vi "Client - JKI SM or SMO.vi"(5 "State Machine Type":enum16{"SMO", "Stand Alone"}(ring)=enum."Stand Alone", 7 "Address":string, 8 "error in (no error)":errorcluster, 11 "RemoteControl":refnum<class "RemoteControl.lvclass">) -> (0 "error out":errorcluster, 3 "RemoteControl out":refnum<class "RemoteControl.lvclass">)   [LabVIEW 2016, in "RemoteControl.lvclass"]
uses:
  RemoteControl.lvclass
  <vilib>/JKI/JKI SMO/SMO/Typedefs/SMOState --Enum.ctl
  C:/Program Files (x86)/National Instruments/LabVIEW 2016/vi.lib/JKI/JKI SMO/SMO/SMO.lvclass
  RemoteControl.lvclass/RemoteControl.ctl
  Typedefs/PrivateEvents--RemoteControl.SendMessageToProcess.ctl
  Typedefs/Message--Cluster.ctl
  <vilib>/JKI/JKI SMO/SMO/SMO.lvclass
panel:
  out "Command out":string
  out "Data out":variant
  in  "Data":variant
  in  "Command":string
  out "# reads":i32
  out "send time":u32
  out "execution time (ms)":u32
  in  "timeout in ms (100)":i32=10
  in  "Send Message":bool
  in  "Stop":bool
  out "message backlog":i32
  out "messages received":i32
  out "messages sent":i32
  in  "Port":u32=6341
  out "SMO State":T1
  # "Client - SM or SMO"
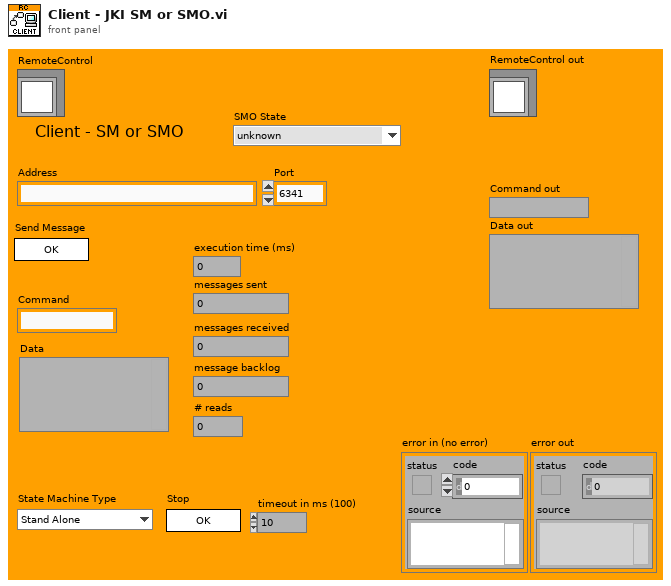
[diagram p1: front panel]
types:
  T1 = typedef "SMO.lvclass/SMOState --Enum.ctl" = enum16{"unknown", "Created", "Started", "Stopped"}
  T2 = enum32{"Invalid", "Standard", "Closed", "Hidden", "Minimized", "Maximized"}
  T3 = enum32{"invalid app kind", "Development System", "Run Time System", "Student Edition", "Embedded LabVIEW", "Evaluation", "Custom"}
  T4 = typedef "RemoteControl.lvclass/PrivateEvents--RemoteControl.SendMessageToProcess.ctl" = cluster{"Message":T5}
  T5 = typedef "RemoteControl.lvclass/Message--Cluster.ctl" = cluster{"Command":string, "Data":variant, "Message ID":i32}
  T6 = cluster{"Core":cluster{"Current VI Reference":refnum<vi>, "Close Panel on Exit?":bool}, "RemoteControl":refnum<class "RemoteControl.lvclass">}
  T7 = cluster{"Current VI Reference":refnum<vi>, "Close Panel on Exit?":bool}
  T8 = typedef "SMO.lvclass/Public Events.ctl" = cluster{"Error":refnum<user-event>, "State":refnum<user-event>, "Reserve State":refnum<user-event>}
  T9 = typedef "RemoteControl.lvclass/PublicEvents--Cluster.ctl" = cluster{"SendMessageFromProcess":refnum<user-event>}
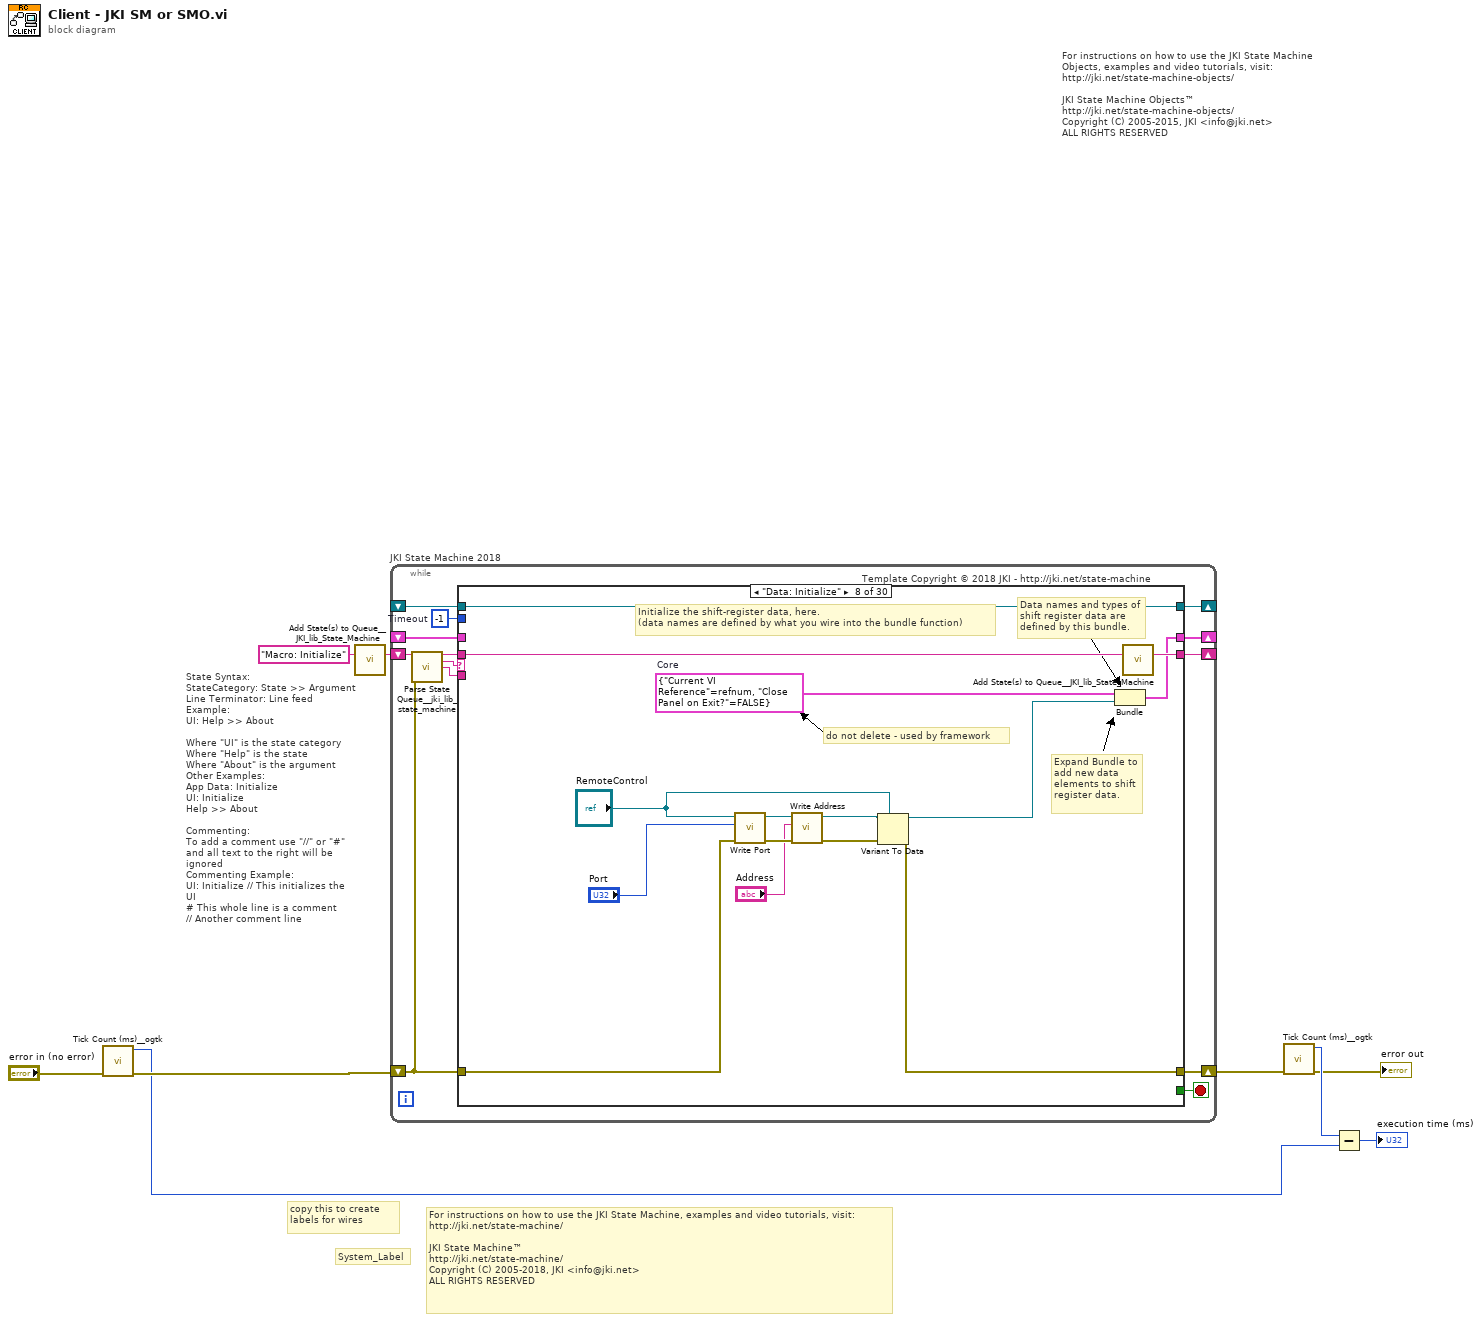
[diagram p0: block diagram]
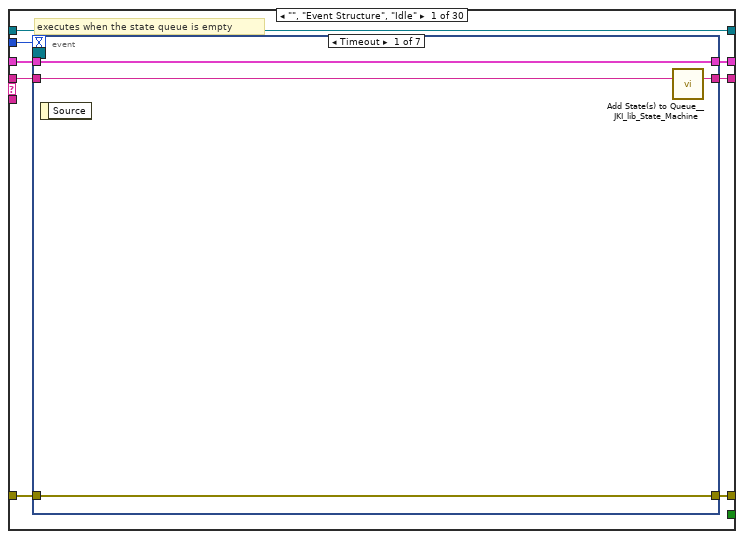
[diagram p2: hidden frame]
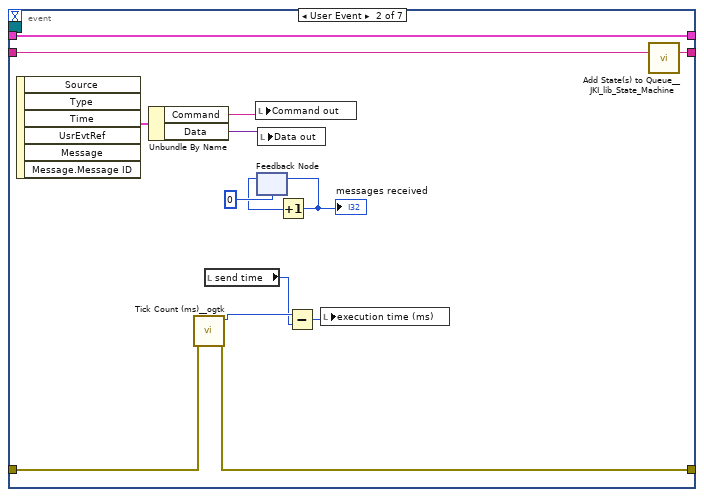
[diagram p3: hidden frame]
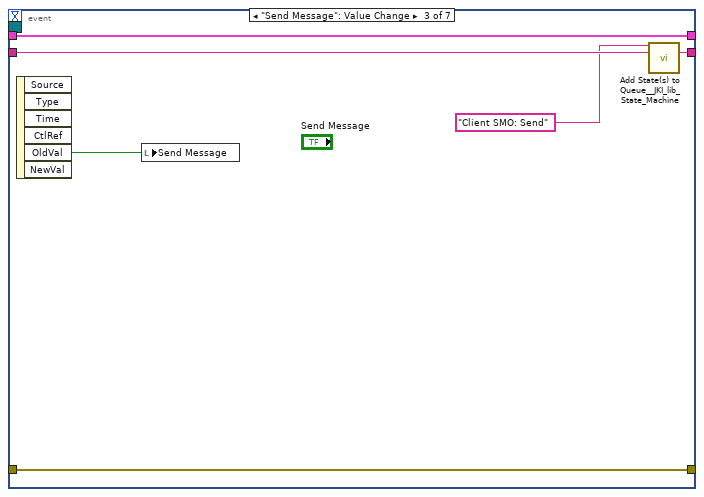
[diagram p4: hidden frame]
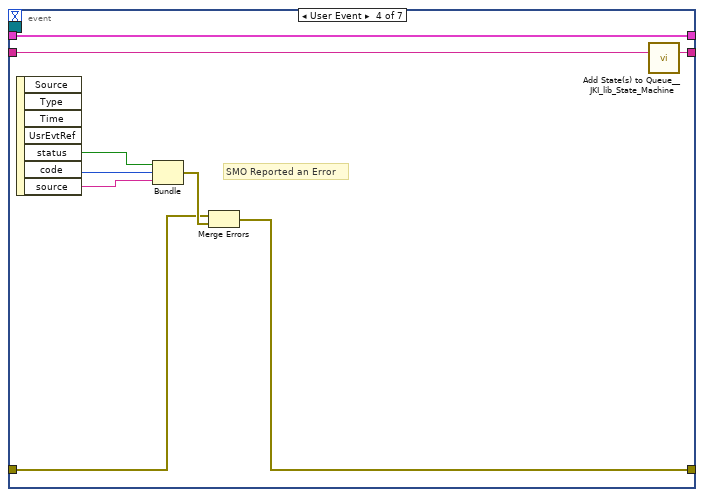
[diagram p5: hidden frame]
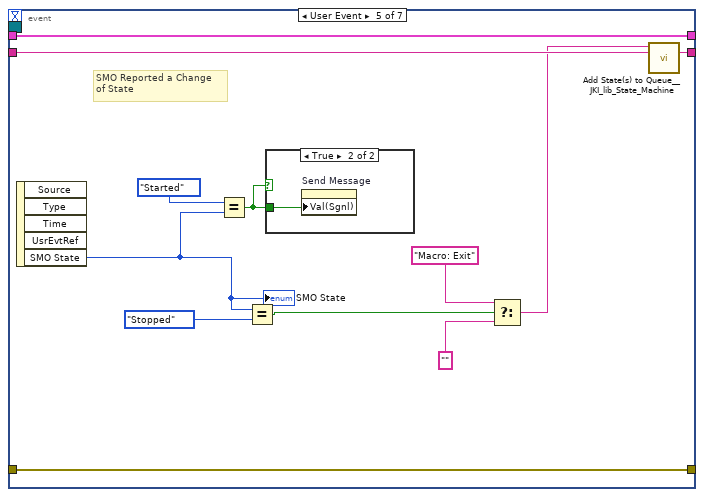
[diagram p6: hidden frame]
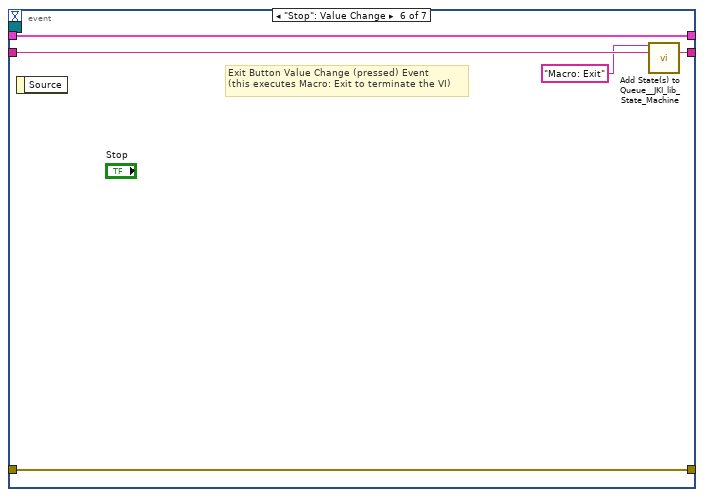
[diagram p8: hidden frame]
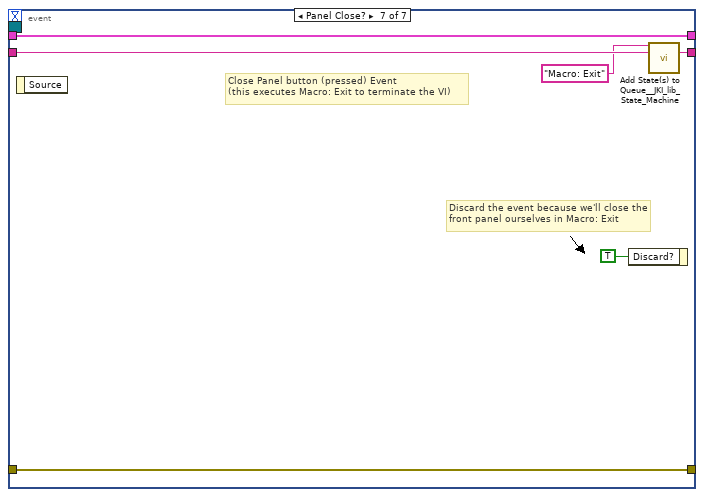
[diagram p9: hidden frame]
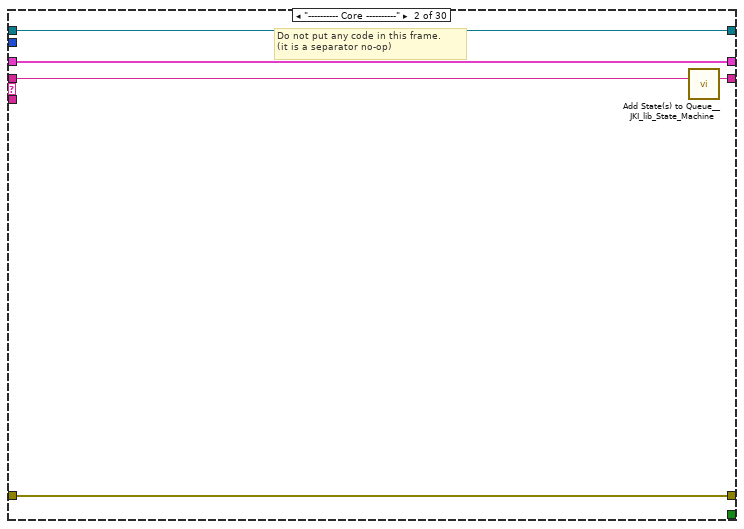
[diagram p10: hidden frame]
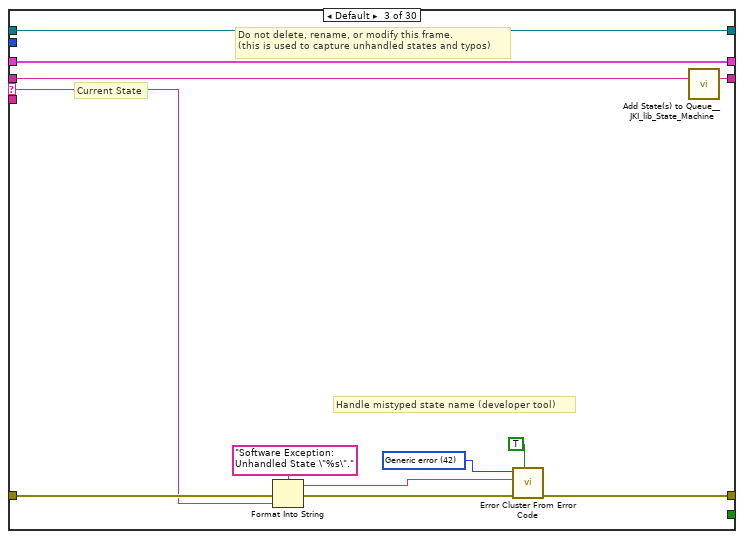
[diagram p11: hidden frame]
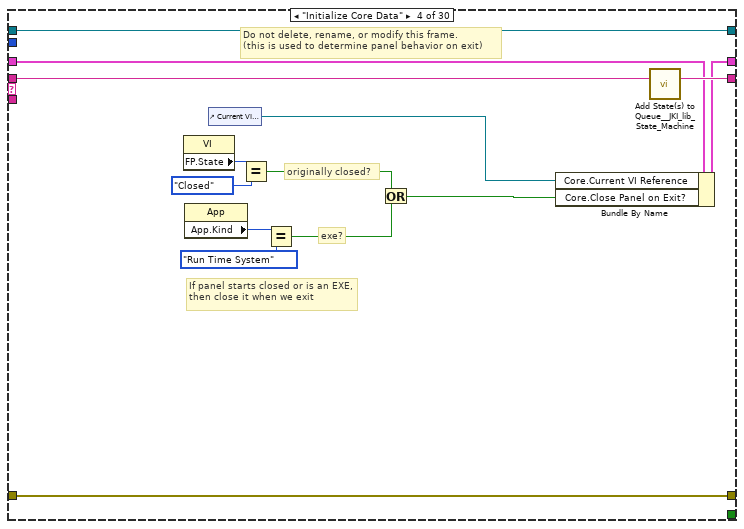
[diagram p12: hidden frame]
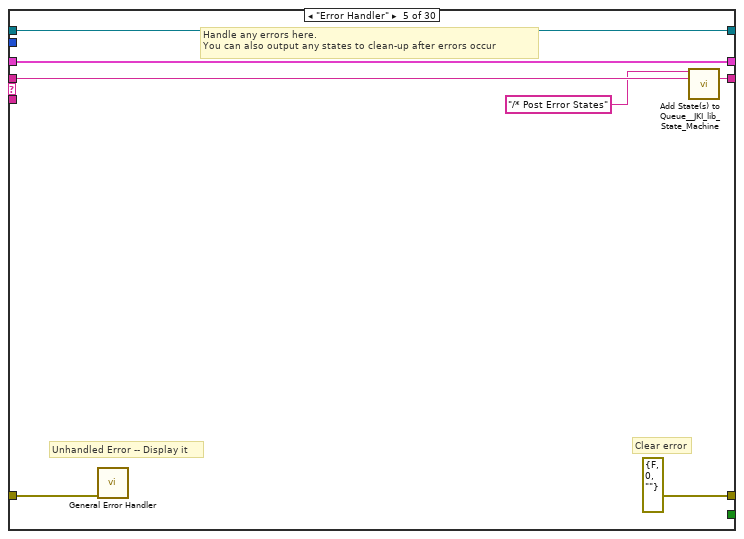
[diagram p13: hidden frame]
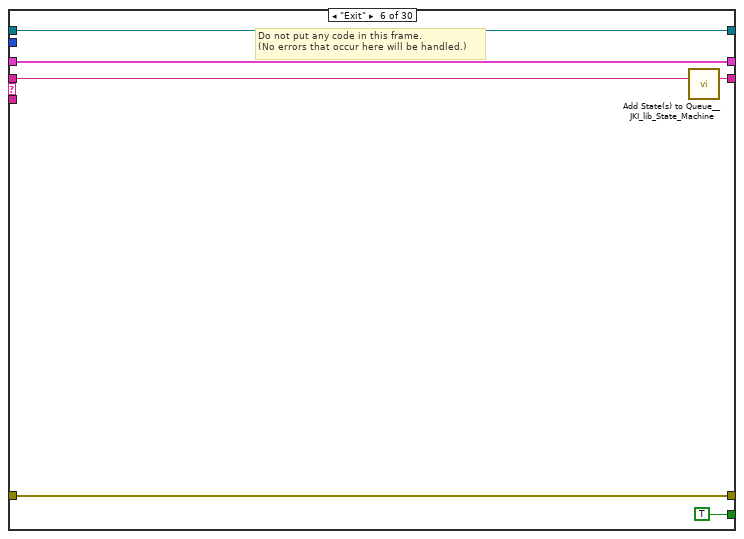
[diagram p14: hidden frame]
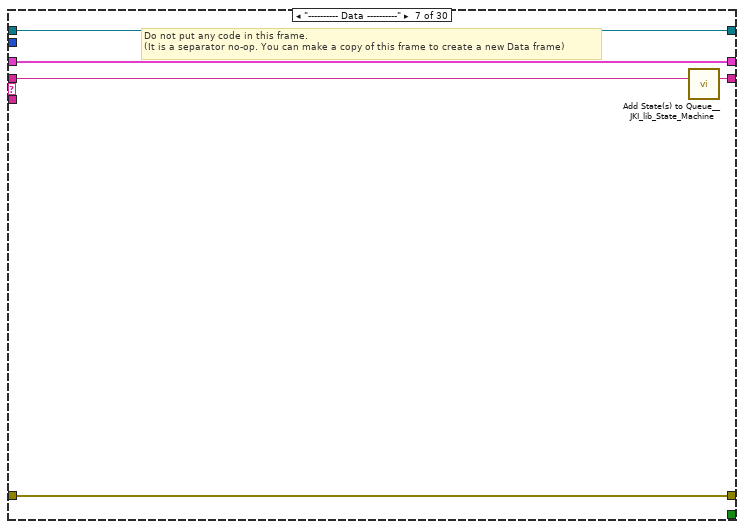
[diagram p15: hidden frame]
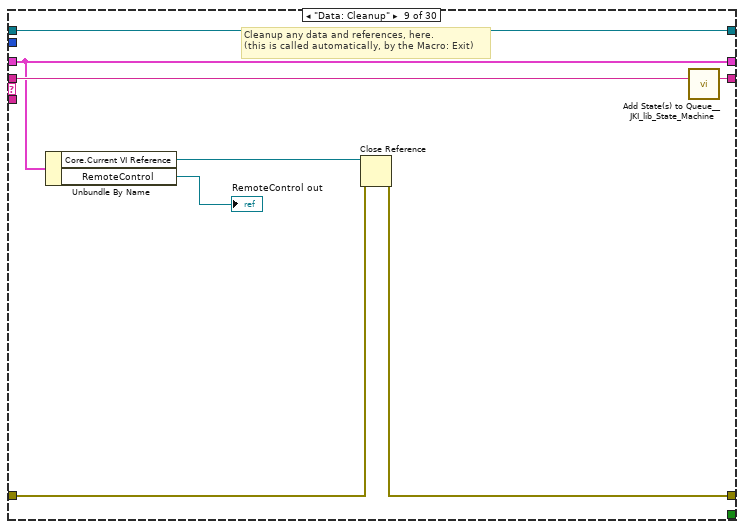
[diagram p16: hidden frame]
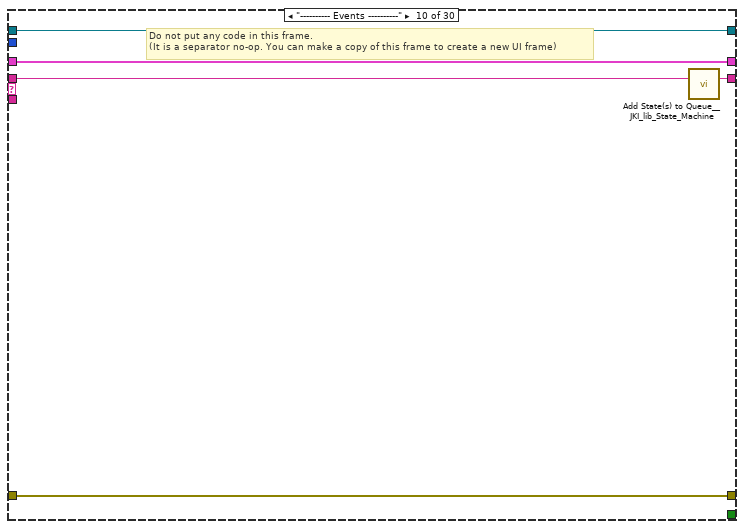
[diagram p17: hidden frame]
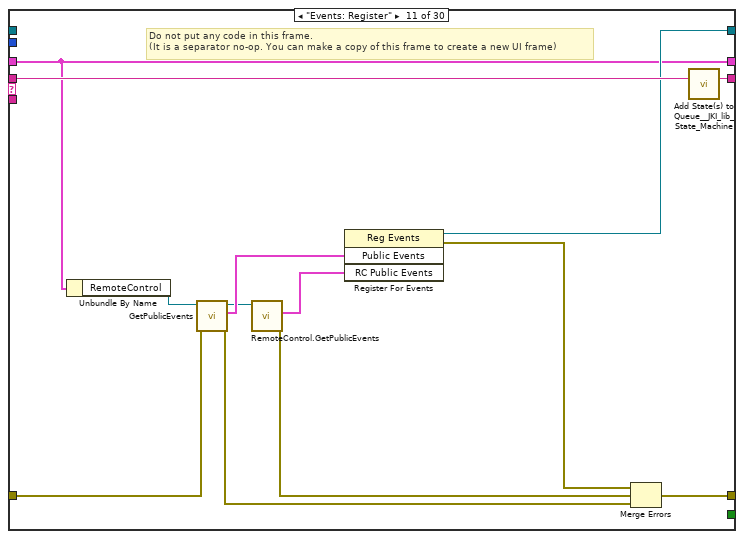
[diagram p18: hidden frame]
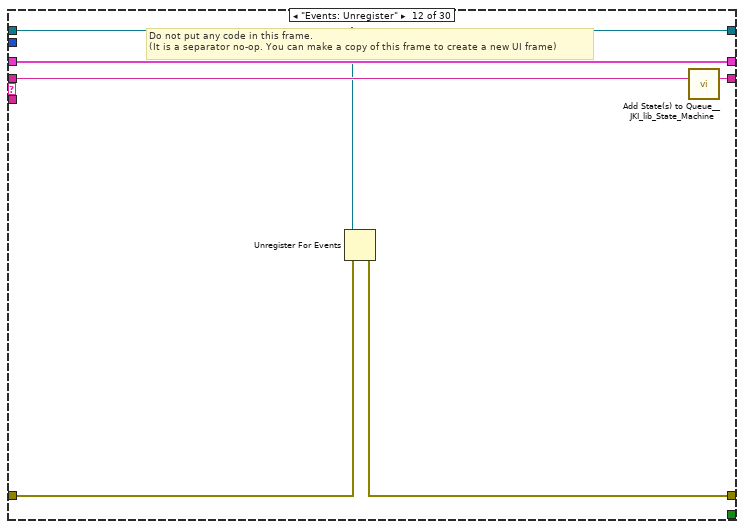
[diagram p19: hidden frame]
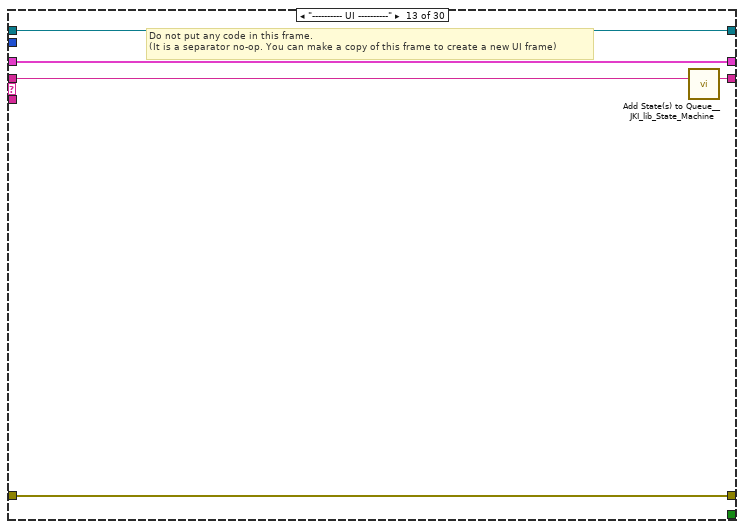
[diagram p20: hidden frame]
diagram:
  # "State Syntax:\nStateCategory: State >> Argument\nLine Terminator: Line feed\nExample:\nUI: Help >> About\n\nWhere \"UI\" is the state category\nWhere \"Help\" is the state\nWhere \"About\" is the argument\nOther Examples:\nApp Data: Initialize\nUI: Initialize\nHelp >> About\n\nCommenting:\nTo add a comment use \"//\" or \"#\" and all text to the right will be ignored\nCommenting Example:\nUI: Initialize // This initializes the UI\n# This whole line is a comment\n// Another comment line"
  # "For instructions on how to use the JKI State Machine, examples and video tutorials, visit:\nhttp://jki.net/state-machine/\n\nJKI State Machine™\nhttp://jki.net/state-machine/\nCopyright (C) 2005-2018, JKI <info@jki.net>\nALL RIGHTS RESERVED"
  # "copy this to create labels for wires"
  # "System_Label"
  # "For instructions on how to use the JKI State Machine Objects, examples and video tutorials, visit:\nhttp://jki.net/state-machine-objects/\n\nJKI State Machine Objects™\nhttp://jki.net/state-machine-objects/\nCopyright (C) 2005-2015, JKI <info@jki.net>\nALL RIGHTS RESERVED"
  n1 = call <userlib>:"Tick Count (ms)__ogtk.vi"("error in (no error)"="error in (no error)") -> ("error out"=w8:errorcluster, "millisecond timer value"=w3:u32)  [unwired: 9 in]
  n2 = call <vilib>:"Add State(s) to Queue__JKI_lib_State_Machine.vi"("State(s) in (\"\")"="Macro: Initialize") -> ("States Out"=w2:string)  [unwired: 14 in]
  n3 = while "JKI State Machine 2018" {
    shift-right: [w15] -> _
    shift-left: _ -> [w14]
    shift-right: [w18] -> w4
    shift-left: w8 -> [w12]
    shift-right: [w17] -> _
    shift-left: w2 -> [w19]
    shift-right: [w11] -> _
    shift-left: _ -> [w10]
    stop <- w16 stop-if-true
    w13 = -1  # Timeout
    # "Template Copyright © 2018 JKI - http://jki.net/state-machine"
    n4 = call <vilib>:"Parse State Queue__jki_lib_state_machine.vi"("State Queue"=w19, "Error In (no error)"=w12) -> ("Remaining States"=w21:string, "Current State"=w22:string, "Arguments"=w20:string)  [unwired: 11 in]
    n5 = case shown="\"Data: Initialize\"" w22 {
      selector: w22 -> [_ _ w94 _ _ _ _ _ _ _ _ _ _ _ _ _ _ _ _ _ _ _ _ _ _ _ _ _ _ _]
      tunnel: w21 -> [w30 w92 w98 w118 w125 w131 w136 w151 w159 w164 w177 w183 w188 w193 w200 w212 w282 w289 w302 w307 w318 w327 w345 w354 w361 w366 w377 w390 w402 w424]
      tunnel: w20 -> [_ _ _ _ _ _ _ _ _ _ _ _ _ _ w195 w206 _ _ _ _ _ _ _ _ _ _ _ _ _ _]
      tunnel: w14 -> [w28 w89 w96 w111 w122 w129 w133 _ w154 w161 w167 w181 w185 w191 w198 w208 w279 w286 w299 w304 w315 w324 w342 w351 w355 w363 w374 w387 w399 w421]
      tunnel: [w27 w90 w100 w115 errorcluster {"status"=FALSE, "code"=0, "source"=""} ("error out") w128 w134 w138 w155 w162 w173 w178 w186 w190 w196 w209 w280 w287 w300 w305 w312 w321 w340 w348 w357 w364 w371 w383 w393 w416] -> w18
      tunnel: w12 -> [w26 w90 w99 w115 w121 w128 w134 w146 w156 w162 w174 w179 w186 w190 w197 w210 w280 w287 w300 w305 w311 w322 w333 w349 w358 w364 w370 w382 w394 w418]
      tunnel: [w29 w91 w97 w117 w124 w130 w135 w150 w158 w163 w176 w182 w187 w192 w199 w211 w281 w288 w301 w306 w317 w326 w344 w353 w360 w365 w376 w389 w401 w423] -> w17
      tunnel: [_ _ _ _ _ TRUE _ _ _ _ _ _ _ _ _ _ _ _ _ _ _ _ _ _ _ _ _ _ _ _] -> w16
      tunnel: [w25 w89 w96 w116 w122 w129 w133 w149 w154 w161 w167 w181 w185 w191 w198 w208 w279 w286 w299 w304 w314 w323 w342 w350 w355 w363 w373 w386 w398 w420] -> w15
      tunnel: w13 -> [w24 _ _ _ _ _ _ _ _ _ _ _ _ _ _ _ _ _ _ _ _ _ _ _ _ _ _ _ _ _]
      tunnel: [w23 w88 w93 w105 w119 w126 w132 w147 w153 w160 w175 w180 w184 w189 w194 w205 w278 w285 w292 w303 w316 w325 w343 w352 w359 w362 w375 w388 w400 w422] -> w11
      tunnel: w10 -> [w23 w88 w93 w105 w119 w126 w132 w147 w153 w160 _ w180 w184 w189 w194 w205 w278 w285 w292 w303 w316 w325 w343 w352 w359 w362 w375 w388 w400 w422]
      frame "", "Event Structure", "Idle" {
        # "executes when the state queue is empty"
        n6 = event shown="[0] Timeout" {
          selector: w23 -> [_ _ _ _ _ _ _]
          dyn-events: _ -> [_ _ _ _ _ _ _]
          timeout: w24 -> [_ _ _ _ _ _ _]
          tunnel: w30 -> [w34 w48 w54 w63 w75 w81 w87]
          tunnel: [w33 w47 w53 w62 w74 w80 w86] -> w29
          tunnel: w28 -> [w31 w46 w51 w61 w72 w78 w84]
          tunnel: [w32 w41 w52 w55 w73 w79 w85] -> w27
          tunnel: w26 -> [w32 w42 w52 w56 w73 w79 w85]
          tunnel: [w31 w46 w51 w61 w72 w78 w84] -> w25
          event Timeout {
            n7 = event-data() -> ()  [unwired: 1 in, 1 out]
            n8 = call <vilib>:"Add State(s) to Queue__JKI_lib_State_Machine.vi"("State(s) in (\"\")"=w34) -> ("States Out"=w33:string)  [unwired: 14 in]
          }
          event User Event {
            n9 = event-data() -> ("Message"=w37:T5)  [unwired: 1 in, 5 out]
            n10 = Unbundle By Name(w37) -> ("Command"=w36:string, "Data"=w35:variant)
            n11 = call <userlib>:"Tick Count (ms)__ogtk.vi"("error in (no error)"=w42) -> ("error out"=w41:errorcluster, "millisecond timer value"=w40:u32)  [unwired: 9 in]
            n12 = local read "send time"() -> (w39:u32)
            n13 = local write "Command out"(w36) -> ()
            n14 = feedback #1(0) -> (w44:i32)
            n15 = local write "Data out"(w35) -> ()
            n16 = Increment(x=w44) -> (x+1=w43:i32)
            "messages received" <- w43
            n17 = feedback-in #1(w43) -> ()
            n18 = Subtract(x=w40, y=w39) -> (x-y=w38:u32)
            n19 = local write "execution time (ms)"(w38) -> ()
            n20 = call <vilib>:"Add State(s) to Queue__JKI_lib_State_Machine.vi"("State(s) in (\"\")"=w48) -> ("States Out"=w47:string)  [unwired: 14 in]
          }
          event "Send Message": Value Change {
            n21 = event-data() -> ("OldVal"=w49:bool)  [unwired: 1 in, 5 out]
            n22 = local write "Send Message"(w49) -> ()
            n23 = call <vilib>:"Add State(s) to Queue__JKI_lib_State_Machine.vi"("State(s) in Front (\"\")"="Client SMO: Send" ("State(s) in Front (\"\")"), "State(s) in (\"\")"=w54) -> ("States Out"=w53:string)  [unwired: 13 in]
          }
          event User Event {
            # "SMO Reported an Error"
            n24 = event-data() -> ("status"=w60:bool, "code"=w59:i32, "source"=w58:string)  [unwired: 1 in, 4 out]
            n25 = Bundle("status"=w60, "code"=w59, "source"=w58) -> (w57:errorcluster)  [unwired: 1 in]
            n26 = Merge Errors(w56, w57) -> (w55:errorcluster)
            n27 = call <vilib>:"Add State(s) to Queue__JKI_lib_State_Machine.vi"("State(s) in (\"\")"=w63) -> ("States Out"=w62:string)  [unwired: 14 in]
          }
          event User Event {
            # "SMO Reported a Change\nof State"
            n28 = event-data() -> ("SMO State"=w66:T1)  [unwired: 1 in, 4 out]
            "SMO State" <- w66
            n29 = Equal?(x=SMOState_--Enum."Started" ("y"), y=w66) -> (x = y?=w64:bool)
            n30 = Equal?(x=w66, y=SMOState_--Enum."Stopped") -> (x = y?=w70:bool)
            n31 = case shown="True" w64 {
              tunnel: w64 -> [_ w76]
              frame False {
              }
              frame True {
                n32 = property on="Send Message" class="Bool (strict)"("Val(Sgnl)"=w76) -> ()  [unwired: 2 in, 2 out]
              }
            }
            n33 = Select(t="Macro: Exit" ("State(s) in Front (\"\")"), s=w70, f="" ("State(s) in Front (\"\")")) -> (s? t:f=w69:string)
            n34 = call <vilib>:"Add State(s) to Queue__JKI_lib_State_Machine.vi"("State(s) in Front (\"\")"=w69, "State(s) in (\"\")"=w75) -> ("States Out"=w74:string)  [unwired: 13 in]
          }
          event "Stop": Value Change {
            # "Exit Button Value Change (pressed) Event\n(this executes Macro: Exit to terminate the VI)"
            n35 = event-data() -> ()  [unwired: 1 in, 1 out]
            n36 = call <vilib>:"Add State(s) to Queue__JKI_lib_State_Machine.vi"("State(s) in Front (\"\")"="Macro: Exit", "State(s) in (\"\")"=w81) -> ("States Out"=w80:string)  [unwired: 13 in]
          }
          event Panel Close? {
            # "Discard the event because we'll close the front panel ourselves in Macro: Exit"
            # "Close Panel button (pressed) Event\n(this executes Macro: Exit to terminate the VI)"
            n37 = event-data() -> ()  [unwired: 1 in, 1 out]
            n38 = event-data("Discard?"=TRUE) -> ()  [unwired: 1 in, 1 out]
            n39 = call <vilib>:"Add State(s) to Queue__JKI_lib_State_Machine.vi"("State(s) in Front (\"\")"="Macro: Exit", "State(s) in (\"\")"=w87) -> ("States Out"=w86:string)  [unwired: 13 in]
          }
        }
      }
      frame "---------- Core ----------" {
        # "Do not put any code in this frame.\n(it is a separator no-op)"
        n40 = call <vilib>:"Add State(s) to Queue__JKI_lib_State_Machine.vi"("State(s) in (\"\")"=w92) -> ("States Out"=w91:string)  [unwired: 14 in]
      }
      frame Default {
        w103 = 42 items=["No error", "Argument error", "Memory is full", "Out of zone", "End of file", "File already open", "Generic file I/O error", "File not found", "File permission error", "Disk is full", "Duplicate path", "Too many files open", "System feature not enabled", "Resource file not found", "Cannot add resource", "Resource not found", "Image not found", "Image memory error", "Pen does not exist", "Config type invalid", "Config token not found", "Config parse error", "Config memory error", "Bad external code format", "Bad external code offset", "External code not present", "Null window", "Destroy window error", "Null menu", "Print aborted", "Bad print record", "Print driver error", "Windows error during printing", "Memory error during printing", "Print dialog error", "Generic print error", "Invalid device refnum", "Device not found", "Device parameter error", "Device unit error", "Cannot open device", "Device call aborted", "Generic error", "Cancelled by user", "Object ID too low", "Object ID too high", "Object not in heap", "Unknown heap", "Unknown object (invalid DefProc)", "Unknown object (DefProc not in table)", "Message out of range", "Invalid (null) method", "Unknown message", "Manager call not supported", "Bad address", "Network operation in progress", "Network operation timed out", "Connection is busy", "Network attribute not supported", "Network error", "Address in use", "System out of memory", "Connection aborted", "Connection refused", "Not connected", "Already connected", "Connection closed", "Initialization error (interapplication manager)", "Bad occurrence", "Wait on unbound occurrence handler", "Occurrence queue overflow", "Datalog type conflict", "Unused", "Unrecognized type (interapplication manager)", "Memory corrupt", "Failed to make temporary DLL", "Old CIN version", "Drag socket not found", "Failed to load drop-object", "Failed to register OLE object", "Failed to release OLE object", "Format specifier type mismatch", "Unknown format specifier", "Too few format specifiers", "Too many format specifiers", "Scan failed", "Newer CIN version", "Error converting to variant", "Runtime menu error", "Password tampered", "Variant attribute not found", "Incompatible variant data type", "Event data is not available", "Event Store is not present", "Occurrence is not found", "Event Queue is not created", "Event info is not available", "Refnum passed is NULL", "Error retrieving Class GUID", "Error retrieving CoClass GUID", "Error retrieving TypeLib GUID.", "Bad built application magic bytes.", "Specific driver is different from the specific driver associated with the Logical Name.", "There is no session opened to the class driver.", "Max Error", "MAX - Error with config objects", "MAX - Error loading configuration", "MAX - Group not supported"]
        # "Current State"
        # "Do not delete, rename, or modify this frame.\n(this is used to capture unhandled states and typos)"
        # "Handle mistyped state name (developer tool)"
        n41 = Format Into String(format string="Software Exception: Unhandled State \"%s\"." ("message"), error in=w99, w94) -> (resulting string=w102:string, error out=w101:errorcluster)  [unwired: 1 in]
        n42 = call <vilib>:"Error Cluster From Error Code.vi"("show call chain? (False)"=TRUE, "error in (no error)"=w101, "error message (\"\")"=w102, "error code (0)"=w103) -> ("error out"=w100:errorcluster)  [unwired: 5 in]
        n43 = call <vilib>:"Add State(s) to Queue__JKI_lib_State_Machine.vi"("State(s) in (\"\")"=w98) -> ("States Out"=w97:string)  [unwired: 14 in]
      }
      frame "Initialize Core Data" {
        # "Do not delete, rename, or modify this frame.\n(this is used to determine panel behavior on exit)"
        # "originally closed?"
        # "exe?"
        # "If panel starts closed or is an EXE, then close it when we exit"
        n44 = property class="VI"() -> ("FP.State"=w108:T2)  [unwired: 2 in, 2 out]
        n45 = property class="App"() -> ("App.Kind"=w114:T3)  [unwired: 2 in, 2 out]
        n46 = control-ref of="Current VI Reference"() -> (w109:refnum<vi>)
        n47 = Equal?(x=w108, y=T2."Closed" ("Front Panel Window:State")) -> (x = y?=w106:bool)
        n48 = Equal?(x=w114, y=T3."Run Time System" ("Application:Kind")) -> (x = y?=w112:bool)
        n49 = Or(x=w106, y=w112) -> (x .or. y?=w110:bool)
        n50 = Bundle By Name(cluster=w111, "Core.Current VI Reference"=w109, "Core.Close Panel on Exit?"=w110) -> (w116:T6)
        n51 = call <vilib>:"Add State(s) to Queue__JKI_lib_State_Machine.vi"("State(s) in (\"\")"=w118) -> ("States Out"=w117:string)  [unwired: 14 in]
      }
      frame "Error Handler" {
        # "Unhandled Error -- Display it"
        # "Handle any errors here.\nYou can also output any states to clean-up after errors occur"
        # "Clear error"
        n52 = call <vilib>:"General Error Handler.vi"("error in (no error)"=w121) -> ()  [unwired: 10 in, 5 out]
        n53 = call <vilib>:"Add State(s) to Queue__JKI_lib_State_Machine.vi"("State(s) in Front (\"\")"="/* Post Error States", "State(s) in (\"\")"=w125) -> ("States Out"=w124:string)  [unwired: 13 in]
      }
      frame "Exit" {
        # "Do not put any code in this frame.\n(No errors that occur here will be handled.)"
        n54 = call <vilib>:"Add State(s) to Queue__JKI_lib_State_Machine.vi"("State(s) in (\"\")"=w131) -> ("States Out"=w130:string)  [unwired: 14 in]
      }
      frame "---------- Data ----------" {
        # "Do not put any code in this frame.\n(It is a separator no-op. You can make a copy of this frame to create a new Data frame)"
        n55 = call <vilib>:"Add State(s) to Queue__JKI_lib_State_Machine.vi"("State(s) in (\"\")"=w136) -> ("States Out"=w135:string)  [unwired: 14 in]
      }
      frame "Data: Initialize" {
        w148 = T7 {"Current VI Reference"=refnum, "Close Panel on Exit?"=FALSE}  # Core
        # "do not delete - used by framework"
        # "Expand Bundle to add new data elements to shift register data."
        # "Data names and types of shift register data are defined by this bundle."
        # "Initialize the shift-register data, here.\n(data names are defined by what you wire into the bundle function)"
        n56 = call-dynamic "Write Port.vi"("error in (no error)"=w146, "Port"="Port", "RemoteControl in"="RemoteControl") -> ("error out"=w145:errorcluster, "RemoteControl out"=w144:refnum<class "RemoteControl.lvclass">)  [unwired: 7 in]
        n57 = call-dynamic "Write Address.vi"("error in (no error)"=w145, "address"="Address", "RemoteControl in"=w144) -> ("error out"=w139:errorcluster, "RemoteControl out"=w140:refnum<class "RemoteControl.lvclass">)  [unwired: 7 in]
        n58 = Variant To Data(error in=w139, type="RemoteControl", Variant=w140) -> (data=w137:refnum<class "RemoteControl.lvclass">, error out=w138:errorcluster)
        n59 = Bundle("Core"=w148, "RemoteControl"=w137) -> (w149:T6)  [unwired: 1 in]
        n60 = call <vilib>:"Add State(s) to Queue__JKI_lib_State_Machine.vi"("State(s) in (\"\")"=w151) -> ("States Out"=w150:string)  [unwired: 14 in]
      }
      frame "Data: Cleanup" {
        # "Cleanup any data and references, here.\n(this is called automatically, by the Macro: Exit)"
        n61 = Unbundle By Name(w154) -> ("Core.Current VI Reference"=w157:refnum<vi>, "RemoteControl"=→"RemoteControl out":refnum<class "RemoteControl.lvclass">)
        n62 = Close Reference(reference=w157, error in (no error)=w156) -> (error out=w155:errorcluster)
        n63 = call <vilib>:"Add State(s) to Queue__JKI_lib_State_Machine.vi"("State(s) in (\"\")"=w159) -> ("States Out"=w158:string)  [unwired: 14 in]
      }
      frame "---------- Events ----------" {
        # "Do not put any code in this frame.\n(It is a separator no-op. You can make a copy of this frame to create a new UI frame)"
        n64 = call <vilib>:"Add State(s) to Queue__JKI_lib_State_Machine.vi"("State(s) in (\"\")"=w164) -> ("States Out"=w163:string)  [unwired: 14 in]
      }
      frame "Events: Register" {
        # "Do not put any code in this frame.\n(It is a separator no-op. You can make a copy of this frame to create a new UI frame)"
        n65 = Unbundle By Name(w167) -> ("RemoteControl"=w166:refnum<class "RemoteControl.lvclass">)
        n66 = call <vilib>:"GetPublicEvents.vi"("error in (no error)"=w174, "SMO"=w166) -> ("error out"=w170:errorcluster, "Public Events"=w172:T8, "SMO out"=w165:refnum<class "RemoteControl.lvclass">)  [unwired: 7 in]
        n67 = call "RemoteControl.GetPublicEvents.vi"("RemoteControl"=w165) -> ("error out"=w169:errorcluster, "RC Public Events"=w171:T9)  [unwired: 8 in, 1 out]
        n68 = register-events(w172, w171) -> (reference out=w175:refnum<event-registration>, error out=w168:errorcluster)  [unwired: 2 in]
        n69 = Merge Errors(w168, w169, w170) -> (w173:errorcluster)
        n70 = call <vilib>:"Add State(s) to Queue__JKI_lib_State_Machine.vi"("State(s) in (\"\")"=w177) -> ("States Out"=w176:string)  [unwired: 14 in]
      }
      frame "Events: Unregister" {
        # "Do not put any code in this frame.\n(It is a separator no-op. You can make a copy of this frame to create a new UI frame)"
        n71 = Unregister For Events(event registration refnum=w180, error in=w179) -> (error out=w178:errorcluster)
        n72 = call <vilib>:"Add State(s) to Queue__JKI_lib_State_Machine.vi"("State(s) in (\"\")"=w183) -> ("States Out"=w182:string)  [unwired: 14 in]
      }
      frame "---------- UI ----------" {
        # "Do not put any code in this frame.\n(It is a separator no-op. You can make a copy of this frame to create a new UI frame)"
        n73 = call <vilib>:"Add State(s) to Queue__JKI_lib_State_Machine.vi"("State(s) in (\"\")"=w188) -> ("States Out"=w187:string)  [unwired: 14 in]
      }
      frame "UI: Initialize" {
        # "Initialize the User Interface, here.\n(this is called automatically, by the Macro: Init)"
        n74 = invoke on="SMO State" class="Enum (strict)" method="Reinit To Default"() -> ()  [unwired: 3 in, 3 out]
        n75 = call <vilib>:"Add State(s) to Queue__JKI_lib_State_Machine.vi"("State(s) in (\"\")"=w193) -> ("States Out"=w192:string)  [unwired: 14 in]
      }
      frame "UI: Cursor Set" {
        # "Argument"
        # "Set and Unset Cursor Busy.\n(Usage: \"UI: Cursor Set >> Busy|Idle\")"
        n76 = case shown="\"Idle\", Default" w195 {
          tunnel: w197 -> [w202 w204]
          tunnel: [w201 w203] -> w196
          frame "Idle", Default {
            n77 = call <vilib>:"Unset Busy.vi"("error in (no error)"=w202) -> ("error out"=w201:errorcluster)  [unwired: 10 in]
          }
          frame "Busy" {
            n78 = call <vilib>:"Set Busy.vi"("error in (no error)"=w204) -> ("error out"=w203:errorcluster)  [unwired: 9 in, 1 out]
          }
        }
        n79 = call <vilib>:"Add State(s) to Queue__JKI_lib_State_Machine.vi"("State(s) in (\"\")"=w200) -> ("States Out"=w199:string)  [unwired: 14 in]
      }
      frame "UI: Front Panel State" {
        # "Argument"
        # "Set Front Panel Open or Closed\n(Usage: \"UI: Front Panel State >> Open|Close\")"
        n80 = Unbundle By Name(w208) -> ("Core.Current VI Reference"=w207:refnum<vi>)
        n81 = case shown="\"Minimize\", \"Minimized\"" w206 {
          tunnel: w210 -> [w218 w233 w244 w257 w270]
          tunnel: [w220 w234 w246 w259 w272] -> w209
          tunnel: w207 -> [w219 w231 w245 w258 w271]
          frame "Open", "Standard", Default {
            w213 = T2."Standard" ("State")
            n82 = property class="VI"(reference=w219, error in=w218) -> (reference out=w216:refnum<vi>, error out=w217:errorcluster, "FP.State"=w215:T2)
            n83 = Not Equal?(x=w215, y=w213) -> (x != y?=w214:bool)
            n84 = case shown="True" w214 {
              tunnel: [w224 w226] -> w220
              tunnel: w217 -> [w223 w226]
              tunnel: w216 -> [w222 _]
              tunnel: w213 -> [w221 _]
              frame True {
                n85 = invoke class="VI" method="FP.Open"(reference=w222, error in=w223, "Activate"=TRUE, "State"=w221) -> (error out=w224:errorcluster)  [unwired: 1 in, 4 out]
              }
              frame False {
              }
            }
          }
          frame "Close", "Closed" {
            n86 = property class="VI"(reference=w231, error in=w233) -> (reference out=w230:refnum<vi>, error out=w232:errorcluster, "FP.State"=w228:T2)
            n87 = Not Equal?(x=w228, y=T2."Closed" ("Front Panel Window:State")) -> (x != y?=w227:bool)
            n88 = case shown="True" w227 {
              tunnel: [w235 w238] -> w234
              tunnel: w232 -> [w235 w237]
              tunnel: w230 -> [_ w236]
              frame False {
              }
              frame True {
                n89 = invoke class="VI" method="FP.Close"(reference=w236, error in=w237) -> (error out=w238:errorcluster)  [unwired: 1 in, 2 out]
              }
            }
          }
          frame "Hidden", "Hide" {
            w239 = T2."Hidden" ("State")
            n90 = property class="VI"(reference=w245, error in=w244) -> (reference out=w242:refnum<vi>, error out=w243:errorcluster, "FP.State"=w241:T2)
            n91 = Not Equal?(x=w241, y=w239) -> (x != y?=w240:bool)
            n92 = case shown="True" w240 {
              tunnel: [w250 w251] -> w246
              tunnel: w243 -> [w249 w251]
              tunnel: w242 -> [w248 _]
              tunnel: w239 -> [w247 _]
              frame True {
                n93 = invoke class="VI" method="FP.Open"(reference=w248, error in=w249, "State"=w247) -> (error out=w250:errorcluster)  [unwired: 2 in, 4 out]
              }
              frame False {
              }
            }
          }
          frame "Minimize", "Minimized" {
            w252 = T2."Minimized" ("State")
            n94 = property class="VI"(reference=w258, error in=w257) -> (reference out=w255:refnum<vi>, error out=w256:errorcluster, "FP.State"=w254:T2)
            n95 = Not Equal?(x=w254, y=w252) -> (x != y?=w253:bool)
            n96 = case shown="True" w253 {
              tunnel: [w263 w264] -> w259
              tunnel: w256 -> [w262 w264]
              tunnel: w255 -> [w261 _]
              tunnel: w252 -> [w260 _]
              frame True {
                n97 = invoke class="VI" method="FP.Open"(reference=w261, error in=w262, "State"=w260) -> (error out=w263:errorcluster)  [unwired: 2 in, 4 out]
              }
              frame False {
              }
            }
          }
          frame "Maximize", "Maximized" {
            w265 = T2."Maximized" ("State")
            n98 = property class="VI"(reference=w271, error in=w270) -> (reference out=w268:refnum<vi>, error out=w269:errorcluster, "FP.State"=w267:T2)
            n99 = Not Equal?(x=w267, y=w265) -> (x != y?=w266:bool)
            n100 = case shown="True" w266 {
              tunnel: [w276 w277] -> w272
              tunnel: w269 -> [w275 w277]
              tunnel: w268 -> [w274 _]
              tunnel: w265 -> [w273 _]
              frame True {
                n101 = invoke class="VI" method="FP.Open"(reference=w274, error in=w275, "State"=w273) -> (error out=w276:errorcluster)  [unwired: 2 in, 4 out]
              }
              frame False {
              }
            }
          }
        }
        n102 = call <vilib>:"Add State(s) to Queue__JKI_lib_State_Machine.vi"("State(s) in (\"\")"=w212) -> ("States Out"=w211:string)  [unwired: 14 in]
      }
      frame "---------- Macro ----------" {
        # "Do not put any code in this frame.\n(It is a separator no-op. You can make a copy of this frame to create a new Macro frame)"
        n103 = call <vilib>:"Add State(s) to Queue__JKI_lib_State_Machine.vi"("State(s) in (\"\")"=w282) -> ("States Out"=w281:string)  [unwired: 14 in]
      }
      frame "Macro: Initialize" {
        # "Initialization Macro\n(This is called once, when the VI starts)"
        n104 = case shown="\"SMO\", Default" "State Machine Type" {
          tunnel: ["Data: Initialize\nInitialize Core Data\nClient SMO: Create\nEvents: Register\nClient SMO: Start\nUI: Initialize\nUI: Front Panel State >> Open" "Data: Initialize\nInitialize Core Data\nClient: Open\nClient: Write\nClient: Read\nClient: Close\nData: Cleanup\nExit"] -> w283
          frame "SMO", Default {
          }
          frame "Stand Alone" {
          }
        }
        n105 = call <vilib>:"Add State(s) to Queue__JKI_lib_State_Machine.vi"("State(s) in Front (\"\")"=w283, "State(s) in (\"\")"=w289) -> ("States Out"=w288:string)  [unwired: 13 in]
      }
      frame "Macro: Exit" {
        # "Exit Macro\n(This is called once, when the VI exits)"
        n106 = Unbundle By Name(w299) -> ("Core.Close Panel on Exit?"=w298:bool)
        n107 = Select(t="UI: Front Panel State >> Close", s=w298, f="") -> (s? t:f=w295:string)
        n108 = call <vilib>:"Add State(s) to Queue__JKI_lib_State_Machine.vi"("State(s) in (\"\")"=w295, "State(s) at Back (\"\")"="Client SMO: Stop\nClient SMO: Destroy\nData: Cleanup\nEvents: Unregister\nExit") -> ("States Out"=w293:string)  [unwired: 13 in]
        n109 = call <vilib>:"Add State(s) to Queue__JKI_lib_State_Machine.vi"("State(s) in Front (\"\")"=w293, "State(s) in (\"\")"=w302) -> ("States Out"=w301:string)  [unwired: 13 in]
      }
      frame "---------- Client SMO ----------" {
        # "Template Separator\n(You can make a copy of, or modify, this frame)"
        n110 = call <vilib>:"Add State(s) to Queue__JKI_lib_State_Machine.vi"("State(s) in (\"\")"=w307) -> ("States Out"=w306:string)  [unwired: 14 in]
      }
      frame "Client SMO: Create" {
        # "Your code here.\n(You can make a copy of, or modify, this frame)"
        n111 = Unbundle By Name(w315) -> ("RemoteControl"=w310:refnum<class "RemoteControl.lvclass">)
        n112 = Unbundle By Name(w310) -> ("address"=w309:string, "Port"=w308:u16)
        n113 = call-dynamic "Create RC Client.vi"("error in (no error)"=w311, "Port"=w308, "address"=w309, "RemoteControl in"=w310) -> ("error out"=w312:errorcluster, "RemoteControl out"=w313:refnum<class "RemoteControl.lvclass">)  [unwired: 6 in]
        n114 = Bundle By Name(cluster=w315, "RemoteControl"=w313) -> (w314:T6)
        n115 = call <vilib>:"Add State(s) to Queue__JKI_lib_State_Machine.vi"("State(s) in (\"\")"=w318) -> ("States Out"=w317:string)  [unwired: 14 in]
      }
      frame "Client SMO: Start" {
        # "Your code here.\n(You can make a copy of, or modify, this frame)"
        n116 = Unbundle By Name(w324) -> ("RemoteControl"=w320:refnum<class "RemoteControl.lvclass">)
        n117 = call <vilib>:"Start.vi"("error in (no error)"=w322, "SMO"=w320) -> ("error out"=w321:errorcluster, "SMO out"=w319:refnum<class "RemoteControl.lvclass">)  [unwired: 8 in]
        n118 = Bundle By Name(cluster=w324, "RemoteControl"=w319) -> (w323:T6)
        n119 = call <vilib>:"Add State(s) to Queue__JKI_lib_State_Machine.vi"("State(s) in (\"\")"=w327) -> ("States Out"=w326:string)  [unwired: 14 in]
      }
      frame "Client SMO: Send" {
        n120 = local read "Command"() -> (w330:string)
        n121 = local read "Data"() -> (w329:variant)
        n122 = Unbundle By Name(w342) -> ("RemoteControl"=w341:refnum<class "RemoteControl.lvclass">)
        n123 = local read "messages received"() -> (w328:i32)
        n124 = call <userlib>:"Tick Count (ms)__ogtk.vi"("error in (no error)"=w333) -> ("error out"=w332:errorcluster, "millisecond timer value"=→"send time":u32)  [unwired: 9 in]
        n125 = Bundle By Name(cluster=T4 {"Message"={"Command"="", "Data"=variant(bool FALSE), "Message ID"=0}} ("SendMessgaeToProcess"), "Message.Command"=w330, "Message.Data"=w329) -> (w338:T4)
        n126 = feedback #2(0) -> (w334:i32)
        n127 = Increment(x=w334) -> (x+1=w336:i32)
        "messages sent" <- w336
        n128 = feedback-in #2(w336) -> ()
        n129 = Subtract(x=w336, y=w328) -> (x-y=→"message backlog":i32)
        n130 = call "RemoteControl.SendMessageToProcess.vi"("error in (no error)"=w332, "SendMessageToProcess"=w338, "RemoteControl"=w341) -> ("error out"=w340:errorcluster)  [unwired: 7 in, 1 out]
        n131 = call <vilib>:"Add State(s) to Queue__JKI_lib_State_Machine.vi"("State(s) in (\"\")"=w345) -> ("States Out"=w344:string)  [unwired: 14 in]
      }
      frame "Client SMO: Stop" {
        # "Your code here.\n(You can make a copy of, or modify, this frame)"
        n132 = Unbundle By Name(w351) -> ("RemoteControl"=w347:refnum<class "RemoteControl.lvclass">)
        n133 = call <vilib>:"Stop.vi"("error in (no error)"=w349, "SMO"=w347) -> ("error out"=w348:errorcluster, "SMO out"=w346:refnum<class "RemoteControl.lvclass">)  [unwired: 8 in]
        n134 = Bundle By Name(cluster=w351, "RemoteControl"=w346) -> (w350:T6)
        n135 = call <vilib>:"Add State(s) to Queue__JKI_lib_State_Machine.vi"("State(s) in (\"\")"=w354) -> ("States Out"=w353:string)  [unwired: 14 in]
      }
      frame "Client SMO: Destroy" {
        # "Your code here.\n(You can make a copy of, or modify, this frame)"
        n136 = Unbundle By Name(w355) -> ("RemoteControl"=w356:refnum<class "RemoteControl.lvclass">)
        n137 = call <vilib>:"Destroy.vi"("error in (no error)"=w358, "SMO"=w356) -> ("error out"=w357:errorcluster)  [unwired: 9 in]
        n138 = call <vilib>:"Add State(s) to Queue__JKI_lib_State_Machine.vi"("State(s) in (\"\")"=w361) -> ("States Out"=w360:string)  [unwired: 14 in]
      }
      frame "---------- Client ----------" {
        # "Template Separator\n(You can make a copy of, or modify, this frame)"
        n139 = call <vilib>:"Add State(s) to Queue__JKI_lib_State_Machine.vi"("State(s) in (\"\")"=w366) -> ("States Out"=w365:string)  [unwired: 14 in]
      }
      frame "Client: Open" {
        # "Your code here.\n(You can make a copy of, or modify, this frame)"
        n140 = Unbundle By Name(w374) -> ("RemoteControl"=w369:refnum<class "RemoteControl.lvclass">)
        n141 = Unbundle By Name(w369) -> ("address"=w368:string, "Port"=w367:u16)
        n142 = call-dynamic "Open Client Connection.vi"("error in (no error)"=w370, "Port"=w367, "address"=w368, "RemoteControl in"=w369) -> ("error out"=w371:errorcluster, "RemoteControl out"=w372:refnum<class "RemoteControl.lvclass">)  [unwired: 6 in]
        n143 = Bundle By Name(cluster=w374, "RemoteControl"=w372) -> (w373:T6)
        n144 = call <vilib>:"Add State(s) to Queue__JKI_lib_State_Machine.vi"("State(s) in (\"\")"=w377) -> ("States Out"=w376:string)  [unwired: 14 in]
      }
      frame "Client: Write" {
        # "Your code here.\n(You can make a copy of, or modify, this frame)"
        n145 = Unbundle By Name(w387) -> ("RemoteControl"=w385:refnum<class "RemoteControl.lvclass">)
        n146 = call <userlib>:"Wait (ms)__ogtk.vi"("error in (no error)"=w382, "milliseconds to wait"=u32 100) -> ("error out"=w381:errorcluster)  [unwired: 8 in, 1 out]
        n147 = call-dynamic "Send Message.vi"("error in (no error)"=w381, "Data"="Data", "Command"="Command", "RemoteControl in"=w385) -> ("error out"=w383:errorcluster, "RemoteControl out"=w384:refnum<class "RemoteControl.lvclass">)  [unwired: 6 in]
        n148 = Bundle By Name(cluster=w387, "RemoteControl"=w384) -> (w386:T6)
        n149 = call <vilib>:"Add State(s) to Queue__JKI_lib_State_Machine.vi"("State(s) in (\"\")"=w390) -> ("States Out"=w389:string)  [unwired: 14 in]
      }
      frame "Client: Read" {
        # "Your code here.\n(You can make a copy of, or modify, this frame)"
        n150 = Unbundle By Name(w399) -> ("RemoteControl"=w397:refnum<class "RemoteControl.lvclass">)
        n151 = while {
          tunnel: w397 -> [w415]
          tunnel: [w414] -> w396
          tunnel: "timeout in ms (100)" -> [w403]
          tunnel: w394 -> [w413]
          tunnel: [w412] -> w393
          tunnel: [w405] -> w391
          tunnel: [w404] -> w392
          i -> [w411]
          stop <- w406 stop-if-true
          n152 = call-dynamic "Read Message.vi"("timeout in ms (100)"=w403, "error in (no error)"=w413, "RemoteControl in"=w415) -> ("error out"=w412:errorcluster, "Data"=w404:variant, "Command"=w405:string, "RemoteControl out"=w414:refnum<class "RemoteControl.lvclass">)  [unwired: 4 in, 1 out]
          n153 = Greater?(x=w411, y=20) -> (0:w408:bool)
          n154 = Empty String/Path?(string/path=w405) -> (empty?=w409:bool)
          n155 = Not(x=w409) -> (.not. x?=w407:bool)
          n156 = Or(x=w407, y=w408) -> (x .or. y?=w406:bool)
          "# reads" <- w411
        }
        "Data out" <- w392
        "Command out" <- w391
        n157 = Bundle By Name(cluster=w399, "RemoteControl"=w396) -> (w398:T6)
        n158 = call <vilib>:"Add State(s) to Queue__JKI_lib_State_Machine.vi"("State(s) in (\"\")"=w402) -> ("States Out"=w401:string)  [unwired: 14 in]
      }
      frame "Client: Close" {
        # "Your code here.\n(You can make a copy of, or modify, this frame)"
        n159 = Unbundle By Name(w421) -> ("RemoteControl"=w419:refnum<class "RemoteControl.lvclass">)
        n160 = call-dynamic "Close Connection.vi"("error in (no error)"=w418, "RemoteControl in"=w419) -> ("error out"=w416:errorcluster, "RemoteControl out"=w417:refnum<class "RemoteControl.lvclass">)  [unwired: 8 in]
        n161 = Bundle By Name(cluster=w421, "RemoteControl"=w417) -> (w420:T6)
        n162 = call <vilib>:"Add State(s) to Queue__JKI_lib_State_Machine.vi"("State(s) in (\"\")"=w424) -> ("States Out"=w423:string)  [unwired: 14 in]
      }
    }
  }
  n163 = call <userlib>:"Tick Count (ms)__ogtk.vi"("error in (no error)"=w4) -> ("error out"=→"error out":errorcluster, "millisecond timer value"=w7:u32)  [unwired: 9 in]
  n164 = Subtract(x=w7, y=w3) -> (x-y=→"execution time (ms)":u32)
